vi "TDS DCPS Set Current.vi"(8 "error in (no error)":errorcluster, 9 "Current":dbl, 10 "Signal InstConfig":string="Regulate", 11 "Address":string) -> (0 "error out":errorcluster)   [LabVIEW 2025, in "Interface Functions.lvlib"]
uses:
  Interface Functions.lvlib
panel:
  # "DCPS Set Current"
  # "Regulate / Trip"
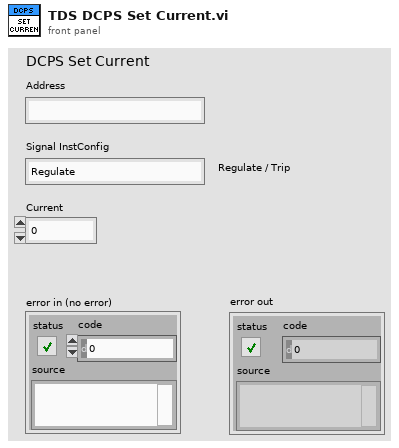
[diagram p1: front panel]
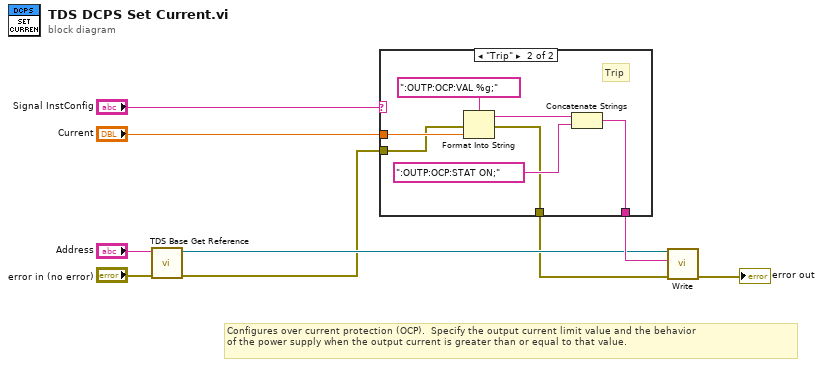
[diagram p0: block diagram]
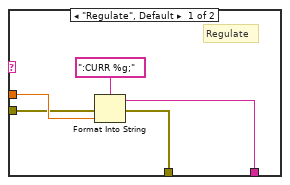
[diagram p2: hidden frame]
diagram:
  # "Configures over current protection (OCP).  Specify the output current limit value and the behavior \nof the power supply when the output current is greater than or equal to that value."
  n1 = call "TDS Base Get Reference.vi"("error in (no error)"="error in (no error)", "Address"="Address") -> ("error out"=w2:errorcluster, "Reference"=w5:refnum<visa-resource-name>)  [unwired: 8 in]
  n2 = case shown="\"Trip\"" "Signal InstConfig" {
    tunnel: "Current" -> [w13 w20]
    tunnel: [w12 w17] -> w7
    tunnel: [w11 w16] -> w3
    tunnel: w2 -> [w10 w15]
    frame "Regulate", Default {
      # "Regulate"
      n3 = Format Into String(format string=":CURR %g;", error in=w10, w13) -> (resulting string=w12:string, error out=w11:errorcluster)  [unwired: 1 in]
    }
    frame "Trip" {
      # "Trip"
      n4 = Format Into String(format string=":OUTP:OCP:VAL %g;", error in=w15, w20) -> (resulting string=w18:string, error out=w16:errorcluster)  [unwired: 1 in]
      n5 = Concatenate Strings(w18, ":OUTP:OCP:STAT ON;") -> (w17:string)
    }
  }
  n6 = call "Write.vi"("error in (no error)"=w3, "Write Buffer (\"\")"=w7, "VISA resource name"=w5) -> ("error out"=→"error out":errorcluster)  [unwired: 7 in, 1 out]
